vi "Refined_Spectra.vi"(4 "Block No":i32=1, 5 "LDA Frequency":sgl=200.0 format="%.2f", 6 "Spectrum input array":dbl[](array[numeric]) format="%.2f", 8 "Sampling frequency":sgl=932.3896 format="%.2f", 11 "X":dbl[](array[numeric])=array[8192 elements]) -> (0 "Spectrum":dbl[](array[numeric]), 3 "Delta f":dbl)   [LabVIEW 2010]
uses:
  <vilib>/Analysis/2dsp.llb/Real FFT.vi
  <vilib>/Analysis/2dsp.llb/Inverse Real FFT.vi
  <vilib>/Analysis/NI_AALPro.lvlib
  <vilib>/Analysis/NI_AALBase.lvlib
panel:
  out "After Filter":dbl[](array[numeric])
  out "First FFT":dbl[](array[numeric])
  out "Waveform Graph 5":dbl[](graph)
  out "Waveform Graph 4":dbl[](graph)
  out "Waveform Graph 3":cluster{sgl, sgl, dbl[]}(graph)
  in  "Dividing Factor":dbl=8.0
  out "Numeric":dbl=2.718281828459045 format="%#_6e"
  out "Waveform Graph":T1(graph)
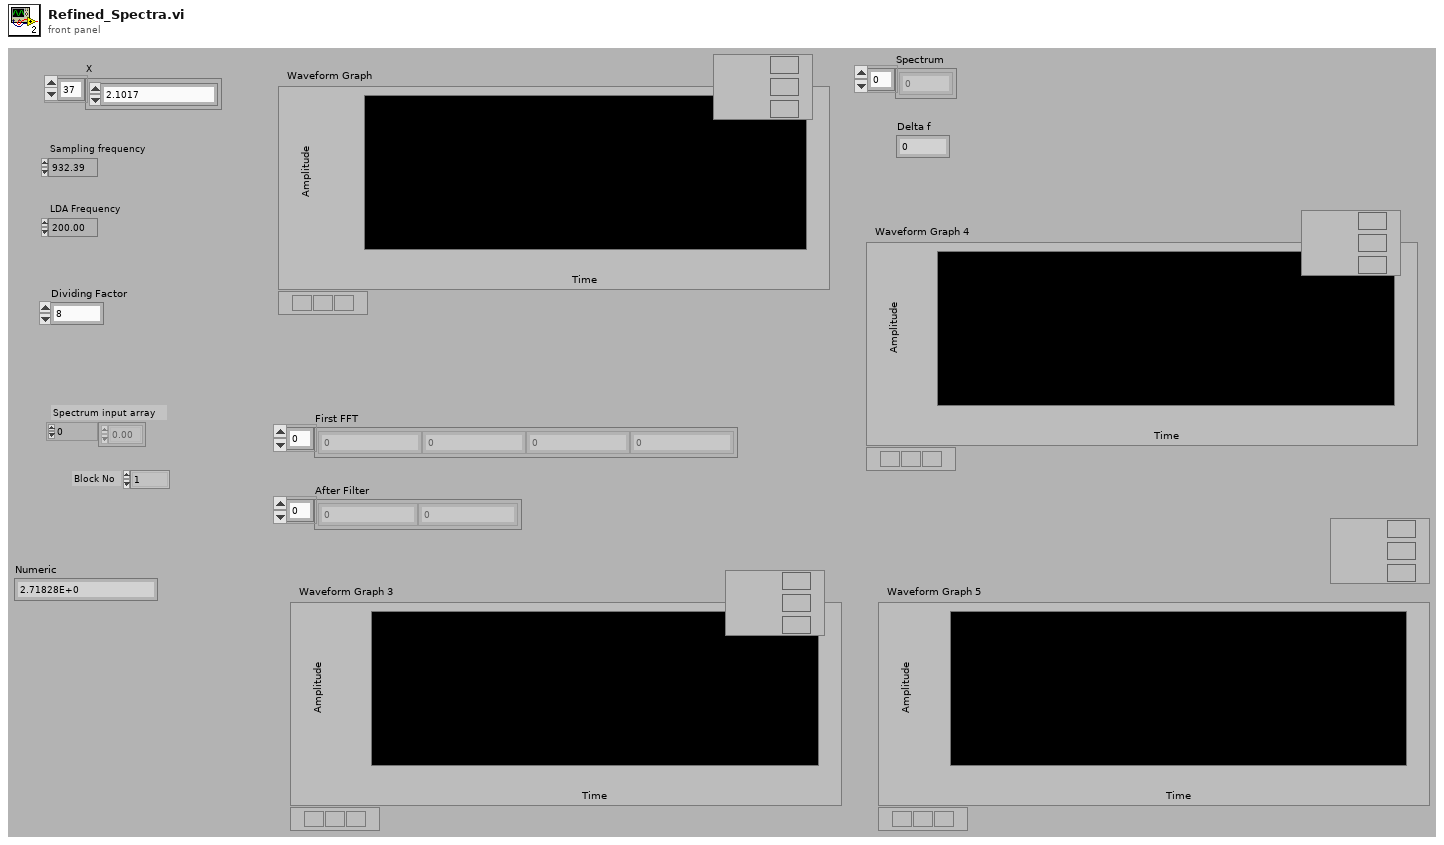
[diagram p1: front panel]
types:
  T1 = cluster{sgl, sgl, "Spectrum output array":dbl[]}[]
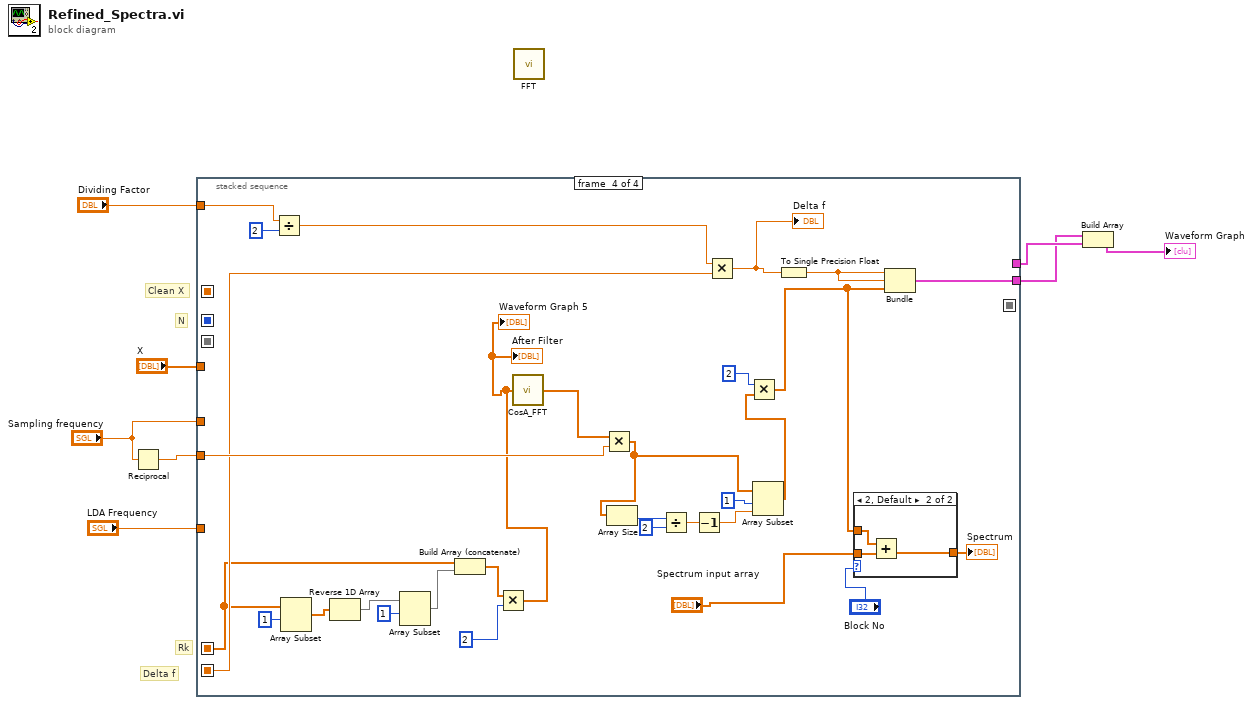
[diagram p0: block diagram]
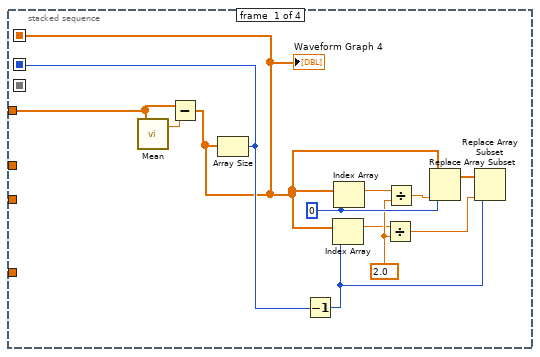
[diagram p2: hidden frame]
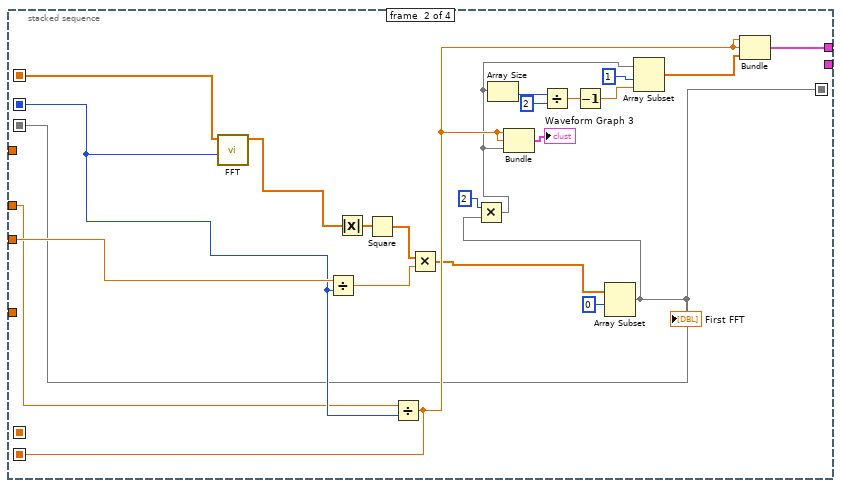
[diagram p3: hidden frame]
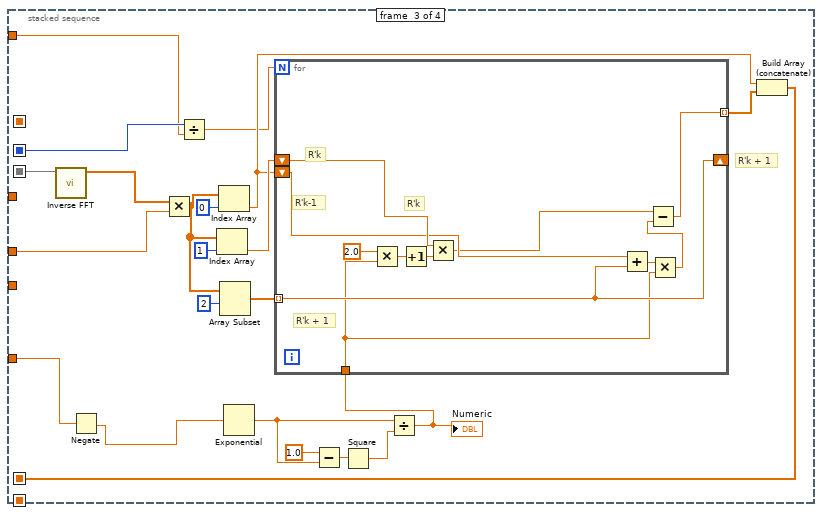
[diagram p4: hidden frame]
diagram:
  # "Delta f"
  # "Rk"
  # "N"
  # "Clean X"
  n1 = Reciprocal(x="Sampling frequency") -> (1/x=w8:sgl)
  n2 = stacked-sequence {
    seq-local: [w9 _ _ _] -> [_ w38 _ _]
    seq-local: [w11 _ _ _] -> [_ w30 w61 _]
    seq-local: [_ w21 _ _] -> [_ _ w64 _]
    seq-local: [_ _ w46 _] -> [_ _ _ w84]
    seq-local: [_ w21 _ _] -> [_ _ _ _]
    seq-local: [_ w26 _ _] -> [_ _ _ w94]
    tunnel: w8 -> [_ w37 _ w105]
    tunnel: "Sampling frequency" -> [_ w27 w62 _]
    tunnel: "LDA Frequency" -> [_ _ w60 _]
    tunnel: [_ w28 _ _] -> w4
    tunnel: "X" -> [w10 _ _ _]
    tunnel: [_ _ _ w98] -> w2
    tunnel: "Dividing Factor" -> [_ _ w43 w97]
    frame #0 {
      w16 = 0
      w15 = 2.0
      n3 = call <vilib>:"Mean.vi"("X"=w10) -> ("mean"=w20:dbl)  [unwired: 1 out]
      n4 = Subtract(x=w10, y=w20) -> (x-y=w9:dbl[])
      "Waveform Graph 4" <- w9
      n5 = Array Size(array=w9) -> (size(s)=w11:i32)
      n6 = Decrement(x=w11) -> (x-1=w19:i32)
      n7 = Index Array(array=w9, index=w19) -> (element=w14:dbl)
      n8 = Index Array(array=w9, index=w16) -> (element=w13:dbl)
      n9 = Divide(x=w14, y=w15) -> (x/y=w18:dbl)
      n10 = Divide(x=w13, y=w15) -> (x/y=w17:dbl)
      n11 = Replace Array Subset(array=w9, new element=w17, index=w16) -> (w12:dbl[])
      n12 = Replace Array Subset(array=w12, new element=w18, index=w19) -> ()  [unwired: 1 out]
    }
    frame #1 {
      n13 = call-poly <vilib>:"FFT.vi"("FFT size"=w30, "X"=w38) -> ("FFT {X}"=w40:cdb[])  [unwired: 8 in, 1 out]
      n14 = Divide(x=w37, y=w30) -> (x/y=w39:sgl)
      n15 = Absolute Value(x=w40) -> (abs(x)=w41:dbl[])
      n16 = Square(x=w41) -> (x^2=w42:dbl[])
      n17 = Divide(x=w27, y=w30) -> (x/y=w26:sgl)
      n18 = Multiply(x=w42, y=w39) -> (x*y=w23:dbl[])
      n19 = Array Subset(array=w23, index=0) -> (w21:dbl[])  [unwired: 1 in]
      "First FFT" <- w21
      n20 = Multiply(x=2, y=w21) -> (x*y=w25:dbl[])
      n21 = Array Size(array=w25) -> (size(s)=w35:i32)
      n22 = Bundle(w26, w26, w25) -> (→"Waveform Graph 3":cluster{sgl, sgl, dbl[]})  [unwired: 1 in]
      n23 = Divide(x=w35, y=2) -> (x/y=w33:dbl)
      n24 = Decrement(x=w33) -> (x-1=w31:dbl)
      n25 = Array Subset(array=w25, index=1, length=w31) -> (w29:dbl[])
      n26 = Bundle(w26, w26, w29) -> (w28:cluster{sgl, sgl, dbl[]})  [unwired: 1 in]
    }
    frame #2 {
      # "R'k + 1"
      n27 = call-poly <vilib>:"Inverse FFT.vi"("FFT {X}"=w64) -> ("X"=w63:dbl[])  [unwired: 9 in, 1 out]
      n28 = Negate(x=w60) -> (-x=w44:sgl)
      n29 = Multiply(x=w63, y=w62) -> (x*y=w52:dbl[])
      n30 = Divide(x=w61, y=w43) -> (x/y=w45:dbl)
      n31 = Index Array(array=w52, index=1) -> (element=w50:dbl)
      n32 = Index Array(array=w52, index=0) -> (element=w48:dbl)
      n33 = Array Subset(array=w52, index=2) -> (w51:dbl[])  [unwired: 1 in]
      n34 = Exponential(1:w44) -> (0:w59:sgl)
      n35 = Subtract(x=sgl 1.0, y=w59) -> (x-y=w57:sgl)
      n36 = Square(x=w57) -> (x^2=w56:sgl)
      n37 = Divide(x=w59, y=w56) -> (x/y=w49:sgl)
      "Numeric" <- w49
      n38 = for {
        N: w45 -> [_]
        shift-right: [w71] -> _
        shift-left: w50 -> [w72]
        shift-left: w48 -> [w70]
        tunnel: w51 -> [w71] mode=indexing
        tunnel: w49 -> [w68]
        tunnel: [w65] -> w47 mode=indexing
        # "R'k"
        # "R'k-1"
        # "R'k"
        # "R'k + 1"
        n39 = Multiply(x=2.0, y=w68) -> (x*y=w74:dbl)
        n40 = Increment(x=w74) -> (x+1=w73:dbl)
        n41 = Multiply(x=w72, y=w73) -> (x*y=w67:dbl)
        n42 = Add(x=w70, y=w71) -> (x+y=w69:dbl)
        n43 = Multiply(x=w69, y=w68) -> (x*y=w66:dbl)
        n44 = Subtract(x=w67, y=w66) -> (x-y=w65:dbl)
      }
      n45 = Build Array (concatenate)(w48, w47) -> (w46:dbl[])
    }
    frame #3 {
      n46 = Divide(x=w97, y=2) -> (x/y=w95:dbl)
      n47 = Array Subset(array=w84, index=1) -> (w81:dbl[])  [unwired: 1 in]
      n48 = Reverse 1D Array(array=w81) -> (reversed array=w80:dbl[])
      n49 = Array Subset(array=w80, index=1) -> (w79:dbl[])  [unwired: 1 in]
      n50 = Build Array (concatenate)(w84, w79) -> (w78:dbl[])
      n51 = Multiply(x=w78, y=2) -> (x*y=w76:dbl[])
      "Waveform Graph 5" <- w76
      "After Filter" <- w76
      n52 = call "CosA_FFT.vi"("Rk"=w76) -> ("Xj"=w85:dbl[])
      n53 = Multiply(x=w85, y=w105) -> (x*y=w102:dbl[])
      n54 = Array Size(array=w102) -> (size(s)=w104:i32)
      n55 = Divide(x=w104, y=2) -> (x/y=w101:dbl)
      n56 = Decrement(x=w101) -> (x-1=w99:dbl)
      n57 = Multiply(x=w95, y=w94) -> (x*y=w86:dbl)
      "Delta f" <- w86
      n58 = Array Subset(array=w102, index=1, length=w99) -> (w91:dbl[])
      n59 = Multiply(x=2, y=w91) -> (x*y=w88:dbl[])
      n60 = To Single Precision Float(number=w86) -> (single precision float=w93:sgl)
      n61 = case shown="2, Default" "Block No" {
        tunnel: [w106 w109] -> w87
        tunnel: w88 -> [w106 w108]
        tunnel: "Spectrum input array" -> [_ w107]
        frame 1 {
        }
        frame 2, Default {
          n62 = Add(x=w108, y=w107) -> (x+y=w109:dbl[])
        }
      }
      "Spectrum" <- w87
      n63 = Bundle(w93, w93, w88) -> (w98:cluster{sgl, sgl, dbl[]})  [unwired: 1 in]
    }
  }
  n64 = call-poly <vilib>:"FFT.vi"() -> ()  [unwired: 10 in, 2 out]
  n65 = Build Array(w2, w4) -> (→"Waveform Graph":cluster{sgl, sgl, dbl[]}[])
